vi "Shutdown.vi"(8 "Error In":errorcluster, 11 "labssh2 Shared Library":path=path "") -> (0 "Error Out":errorcluster)   [LabVIEW 2017, in "LabSSH2.lvlib"]
uses:
  LabSSH2.lvlib
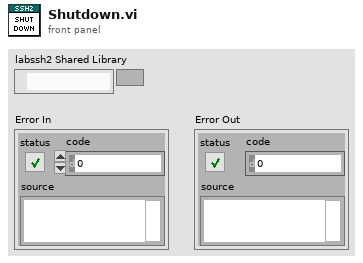
[diagram p1: front panel]
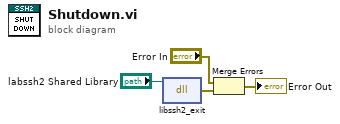
[diagram p0: block diagram]
diagram:
  n1 = dll-call lib="D:/Users/cfield/Code/Field R&D Services/SSH/LabSSH2/LabVIEW/trunk/src/LabSSH2/Private/labssh2.*" fn="libssh2_exit"(path in="labssh2 Shared Library") -> (error out=w2:errorcluster)  [unwired: 3 in, 1 out]
  n2 = Merge Errors("Error In", w2) -> (→"Error Out":errorcluster)
